vi "zern2slopes_test.vi"() -> ()   [LabVIEW 2018]
uses:
  <userlib>/WaveKit.lib/Classes/ModalCoef/ModalCoef.lvclass
  <userlib>/WaveKit.lib/Controls/WavefrontModalReconstructionType.ctl
  <userlib>/WaveKit.lib/Controls/ZernikeModalPrefs.ctl
  <userlib>/WaveKit.lib/Controls/ZernikeProjectionPupilSetup.ctl
  <userlib>/WaveKit.lib/Controls/Point2Df.ctl
  <userlib>/WaveKit.lib/Controls/CircularPupilDetectionParams.ctl
  <userlib>/WaveKit.lib/Controls/PupilDetectionOption.ctl
  <userlib>/WaveKit.lib/Controls/CircularAutoDetectionOptions.ctl
  <userlib>/WaveKit.lib/Controls/PupilDetectionMode.ctl
  <userlib>/WaveKit.lib/Controls/HasoSlopes.lvclass
  <userlib>/WaveKit.lib/Controls/Pupil.lvclass
  <userlib>/WaveKit.lib/Classes/HasoData/HasoData.lvclass
  <userlib>/WaveKit.lib/Classes/ComputePhaseSet/ComputePhaseSet.lvclass
  <userlib>/WaveKit.lib/Controls/WavefrontReconstructionMode.ctl
  <vilib>/Analysis/1siggen.llb/Ramp Pattern by Delta.vi
  <userlib>/WaveKit.lib/Classes/Phase/Phase.lvclass
  <vilib>/Analysis/NI_AALBase.lvlib
panel:
  in  "Output folder":path=path "D:/Data/20200122_Test"
  in  "Output file name":string="test.dat"
  out "Phase values":sgl[][](graph)
  out "Number of Coefficients":i32
  out "Zernike pupil":i32[][](graph)
  out "Zernike Coefficients":sgl[](graph)
  out "Zern index":i32[](array[numeric]) min=1 max=32
  in  "Initial haso file":path=path "D:/SystemAlignment/system_aberration_residual_20191015.has"
  out "Haso pupil":i32[][](graph)
  out "error out":errorcluster
  in  "error in (no error)":errorcluster
  in  "Input coef":sgl[](array[numeric])
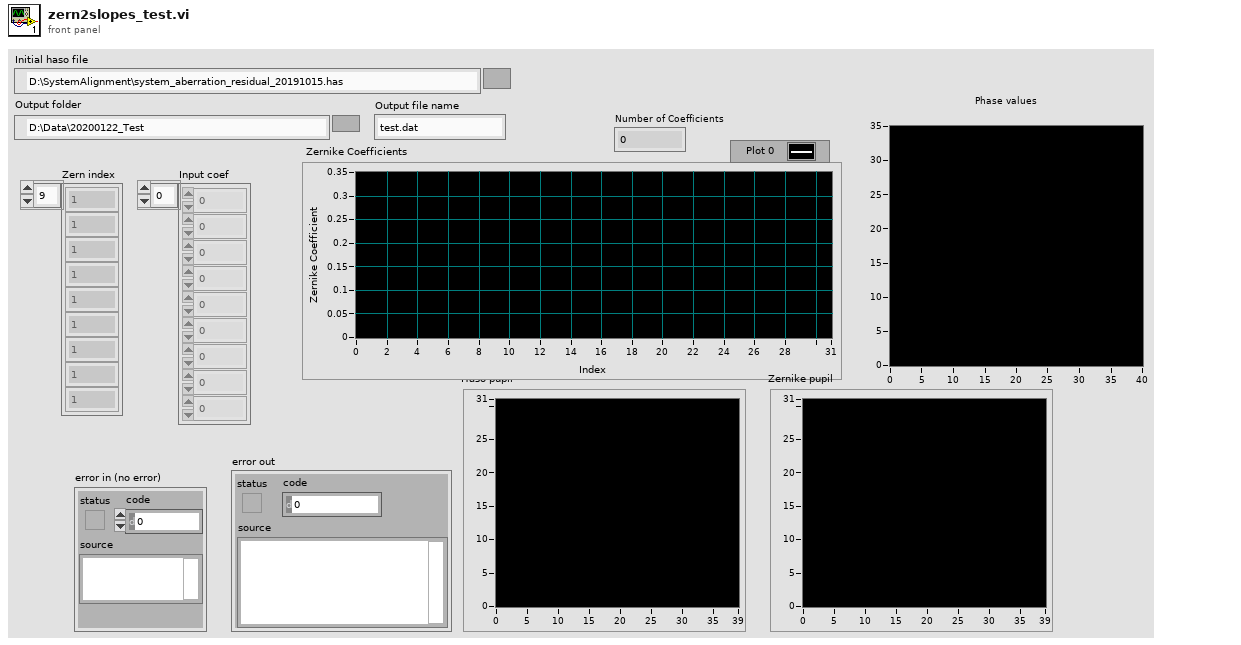
[diagram p1: front panel]
types:
  T1 = typedef "WavefrontReconstructionMode.ctl" = enum16{"None", "Modal_Legendre", "Modal_Zernike", "Zonal", "Modal_Zonal_Zernike", "Modal_Zonal_Legendre"}
  T2 = typedef "CircularPupilDetectionParams.ctl" = cluster{"PupilDetectionOption":T3, "AutoDetectionOption":T4, "PupilDetectionMode":T5, "CentralOccultationDetection":bool}
  T3 = typedef "PupilDetectionOption.ctl" = enum16{"Manual", "Automatic"}
  T4 = typedef "CircularAutoDetectionOptions.ctl" = enum16{"manual_radius_auto_center", "manual_center_auto_radius", "auto_radius_auto_center"}
  T5 = typedef "PupilDetectionMode.ctl" = enum16{"inscribed", "circumscribed"}
  T6 = typedef "ZernikeModalPrefs.ctl" = cluster{"Number of coefficients":u32, "Filtered coefficients":u32[], "RMS Zernike normalization":bool, "CircularProjectionPupilDimensions":T7}
  T7 = typedef "ZernikeProjectionPupilSetup.ctl" = cluster{"Pupil center_sspp":T8, "Pupil radius_sspp":sgl}
  T8 = typedef "Point2Df.ctl" = cluster{"X":sgl, "Y":sgl}
  T9 = typedef "WavefrontModalReconstructionType.ctl" = enum16{"Legendre", "Zernike"}
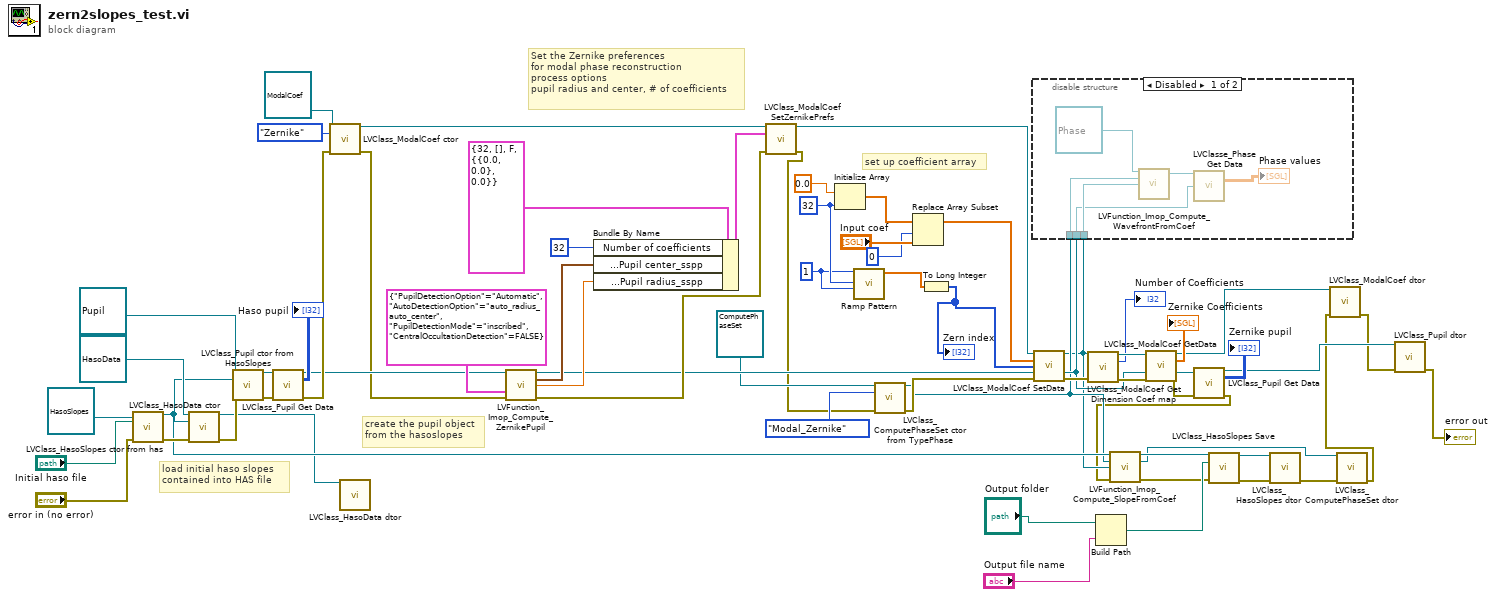
[diagram p0: block diagram]
diagram:
  w2 = 1
  w3 = 32
  # "create the pupil object\nfrom the hasoslopes"
  # "load initial haso slopes\ncontained into HAS file"
  # "Set the Zernike preferences\nfor modal phase reconstruction\nprocess options\npupil radius and center, # of coefficients"
  # "set up coefficient array"
  n1 = call <userlib>:"LVClass_HasoSlopes ctor from has.vi"("HasoSlopes in"=refnum<class "HasoSlopes.lvclass"> refnum, ".has path"="Initial haso file", "error in (no error)"="error in (no error)") -> ("HasoSlopes out"=w23:refnum<class "HasoSlopes.lvclass">, "error out"=w52:errorcluster)  [unwired: 11 in]
  n2 = call <userlib>:"LVClass_HasoData ctor.vi"("HasoData in"=refnum<class "HasoData.lvclass"> refnum, "HasoSlopes.lvclass"=w23, "error in (no error)"=w52) -> ("HasoData out"=w11:refnum<class "HasoData.lvclass">, "error out"=w51:errorcluster)  [unwired: 11 in]
  n3 = call <userlib>:"LVClass_Pupil ctor from HasoSlopes.vi"("Pupil in"=refnum<class "Pupil.lvclass"> refnum, "HasoSlopes.lvclass"=w23, "error in (no error)"=w51) -> ("Pupil out"=w50:refnum<class "Pupil.lvclass">, "error out"=w49:errorcluster)  [unwired: 11 in]
  n4 = call <userlib>:"LVClass_Pupil Get Data.vi"("Pupil in"=w50, "error in (no error)"=w49) -> ("Pupil out"=w44:refnum<class "Pupil.lvclass">, "Data"=→"Haso pupil":i32[][], "error out"=w47:errorcluster)  [unwired: 11 in]
  n5 = call <userlib>:"LVClass_ModalCoef ctor.vi"("ModalCoef in"=refnum<class "ModalCoef.lvclass"> refnum, "TypePhase"=WavefrontModalReconstructionType."Zernike", "error in (no error)"=w47) -> ("ModalCoef out"=w60:refnum<class "ModalCoef.lvclass">, "error out"=w43:errorcluster)  [unwired: 11 in]
  n6 = call <userlib>:"LVClass_HasoData dtor.vi"("HasoData in"=w11) -> ()  [unwired: 13 in, 2 out]
  n7 = call <userlib>:"LVFunction_Imop_Compute_ZernikePupil.vi"("Pupil.lvclass"=w44, "CircularPupilDetectionParams"=T2 {"PupilDetectionOption"=enum."Automatic", "AutoDetectionOption"=enum."auto_radius_auto_center", "PupilDetectionMode"=enum."inscribed", "CentralOccultationDetection"=FALSE}, "error in"=w43) -> ("Pupil.lvclass"=w39:refnum<class "Pupil.lvclass">, "center"=w56:T8, "radius"=w57:sgl, "error out"=w40:errorcluster)  [unwired: 9 in]
  n8 = Bundle By Name(cluster=T6 {"Number of coefficients"=32, "Filtered coefficients"=[], "RMS Zernike normalization"=FALSE, "CircularProjectionPupilDimensions"={"Pupil center_sspp"={"X"=0.0, "Y"=0.0}, "Pupil radius_sspp"=0.0}} ("ZernikeModalPrefs"), "Number of coefficients"=u32 32, "CircularProjectionPupilDimensions.Pupil center_sspp"=w56, "CircularProjectionPupilDimensions.Pupil radius_sspp"=w57) -> (w62:T6)
  n9 = call <userlib>:"LVClass_ModalCoef SetZernikePrefs.vi"("ModalCoef in"=w60, "ZernikeModalPrefs"=w62, "error in (no error)"=w40) -> ("ModalCoef out"=w38:refnum<class "ModalCoef.lvclass">, "error out"=w34:errorcluster)  [unwired: 11 in]
  n10 = Initialize Array(0.0, w3) -> (w42:dbl[])
  n11 = call-poly <vilib>:"Ramp Pattern.vi"("start"=w2, "end"=w3, "delta"=w2) -> ("Ramp Pattern"=w4:dbl[])  [unwired: 6 in, 2 out]
  n12 = call <userlib>:"LVClass_ComputePhaseSet ctor from TypePhase.vi"("ComputePhaseSet in"=refnum<class "ComputePhaseSet.lvclass"> refnum, "TypePhase"=WavefrontReconstructionMode."Modal_Zernike", "error in (no error)"=w34) -> ("ComputePhaseSet out"=w22:refnum<class "ComputePhaseSet.lvclass">, "error out"=w33:errorcluster)  [unwired: 11 in]
  n13 = Replace Array Subset(array=w42, new element="Input coef", index=0) -> (w37:dbl[])
  n14 = To Long Integer(number=w4) -> (32bit integer=w1:i32[])
  "Zern index" <- w1
  n15 = call <userlib>:"LVClass_ModalCoef SetData.vi"("ModalCoef in"=w38, "coef"=w37, "index"=w1, "Pupil.lvclass"=w39, "error in (no error)"=w33) -> ("ModalCoef out"=w21:refnum<class "ModalCoef.lvclass">, "Pupil (dup)"=w24:refnum<class "Pupil.lvclass">, "error out"=w26:errorcluster)  [unwired: 7 in, 1 out]
  n16 = disable-structure shown="Disabled" {
    disable-tunnel: w22 -> [w71 _]
    disable-tunnel: w21 -> [w70 _]
    disable-tunnel: w24 -> [w68 _]
    frame Disabled {
      n17 = call <userlib>:"LVFunction_Imop_Compute_WavefrontFromCoef.vi"("Phase"=refnum<class "Phase.lvclass"> refnum ("Phase in"), "ComputePhaseSet"=w71, "ModalCoef"=w70) -> ("Phase"=w67:refnum<class "Phase.lvclass">)  [unwired: 9 in, 3 out]
      n18 = call <userlib>:"LVClasse_Phase Get Data.vi"("Phase in"=w67, "Pupil"=w68) -> ("data"=→"Phase values":sgl[][])  [unwired: 10 in, 3 out]
    }
    frame Enabled {
    }
  }
  n19 = call <userlib>:"LVClass_ModalCoef Get Dimension Coef map.vi"("ModalCoef in"=w21, "error in (no error)"=w26) -> ("ModalCoef out"=w32:refnum<class "ModalCoef.lvclass">, "# of coef"=→"Number of Coefficients":i32, "error out"=w31:errorcluster)  [unwired: 11 in]
  n20 = Build Path(base path="Output folder", name or relative path="Output file name") -> (appended path=w17:path)
  n21 = call <userlib>:"LVClass_ModalCoef GetData.vi"("ModalCoef in"=w32, "Pupil.lvclass"=w24, "error in (no error)"=w31) -> ("ModalCoef out"=w9:refnum<class "ModalCoef.lvclass">, "coef"=→"Zernike Coefficients":sgl[], "Pupil.lvclass (dup)"=w29:refnum<class "Pupil.lvclass">, "error out"=w28:errorcluster)  [unwired: 8 in, 1 out]
  n22 = call <userlib>:"LVClass_Pupil Get Data.vi"("Pupil in"=w29, "error in (no error)"=w28) -> ("Pupil out"=w10:refnum<class "Pupil.lvclass">, "Data"=→"Zernike pupil":i32[][], "error out"=w6:errorcluster)  [unwired: 11 in]
  n23 = call <userlib>:"LVFunction_Imop_Compute_SlopeFromCoef.vi"("HasoSlopes.lvclass"=w23, "ComputePhaseSet"=w22, "ModalCoef.lvclass"=w21, "error IO"=w6) -> ("HasoSlopes.lvclass"=w18:refnum<class "HasoSlopes.lvclass">, "ComputePhaseSet (dup)"=w13:refnum<class "ComputePhaseSet.lvclass">, "error IO out"=w15:errorcluster)  [unwired: 8 in, 1 out]
  n24 = call <userlib>:"LVClass_HasoSlopes Save.vi"("HasoSlopes in"=w18, "path"=w17, "error in (no error)"=w15) -> ("HasoSlopes out"=w16:refnum<class "HasoSlopes.lvclass">, "error out"=w14:errorcluster)  [unwired: 11 in]
  n25 = call <userlib>:"LVClass_HasoSlopes dtor.vi"("HasoSlopes in"=w16, "error in (no error)"=w14) -> ("error out"=w12:errorcluster)  [unwired: 12 in, 1 out]
  n26 = call <userlib>:"LVClass_ComputePhaseSet dtor.vi"("ComputePhaseSet in"=w13, "error in (no error)"=w12) -> ("error out"=w5:errorcluster)  [unwired: 12 in, 1 out]
  n27 = call <userlib>:"LVClass_ModalCoef dtor.vi"("ModalCoef in"=w9, "error in (no error)"=w5) -> ("error out"=w8:errorcluster)  [unwired: 12 in, 1 out]
  n28 = call <userlib>:"LVClass_Pupil dtor.vi"("Pupil in"=w10, "error in (no error)"=w8) -> ("error out"=→"error out":errorcluster)  [unwired: 12 in, 1 out]
